vi "test Process Records.vi"(8 "error in":errorcluster, 11 "TestCase in":refnum<class "Engine.lvclass">) -> (0 "error out":errorcluster, 3 "TestCase out":refnum<class "Engine.lvclass">)   [LabVIEW 2023, in "Engine.lvclass"]
uses:
  Engine.lvclass
  Engine.lvclass/Engine.ctl
  <vilib>/addons/_JKI Toolkits/VI Tester/TestCase.llb/TestCase.lvclass
  <instrlib>/BTICardLib/Public/Controls/429 Record.ctl
  <instrlib>/BTICardLib/BTICardLV.lvlib
  <vilib>/NI VeriStand/Custom Device API/Data Reference.ctl
  <vilib>/NI VeriStand/Custom Device API/Custom Device API.lvlib
  <vilib>/NI VeriStand/Custom Device API/Custom Device Item Ref.ctl
  Shared/Transfer Type.ctl
  <vilib>/NI/NI VeriStand Encoding and Decoding/Encoding.ctl
  <vilib>/NI/NI VeriStand Encoding and Decoding/Encoding and Decoding.lvlib
  Shared/Parameter Definition.ctl
  Shared/RT Parameters.ctl
  Shared/Label.ctl
  Shared/RT Label Settings.ctl
  Shared/RT Hardware Channel Settings.ctl
  Shared/Map of Identifiers to Indexes.ctl
  Engine/Custom Device/Custom Device.lvlib
  C:/Program Files/National Instruments/LabVIEW 2023/vi.lib/addons/_JKI Toolkits/VI Tester/TestCase.llb/TestCase.lvclass
  C:/dev/niveristand-ballard-arinc429-custom-device/Source/Custom Device Support/Tests/Unit/Execution/Engine/Engine.lvclass
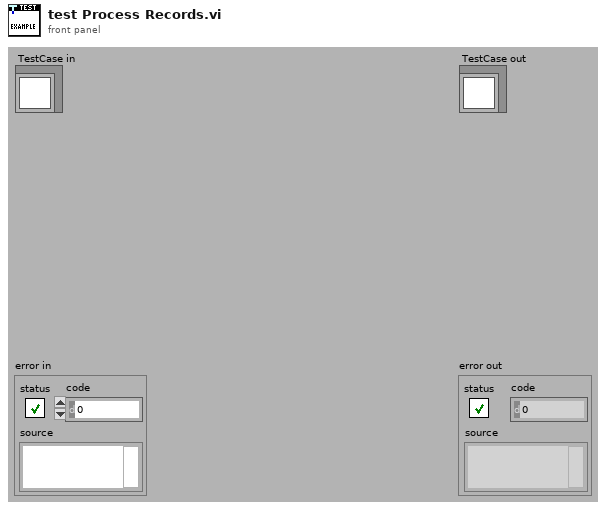
[diagram p1: front panel]
types:
  T1 = typedef "Map of Identifiers to Indexes.ctl" = map{u32, cluster{"channel index":i32, "label index":i32, "start index":i32, "parameters":i32, "timestamp index":i32}}
  T2 = typedef "BTICardLV.lvlib/429 Record.ctl" = cluster{"type":u16, "count":u16, "timestamp":u32, "msgact":u16, "decgap":u16, "data":u32, "timestamph":u32}
  T3 = typedef "RT Hardware Channel Settings.ctl" = cluster{"channel #":u16, "channel handle":u64, "labels settings for RT":T4[]}
  T4 = typedef "RT Label Settings.ctl" = cluster{"Name":string, "xmlName":string, "label":T5, "transfer period":u32, "SDI_Enabled":bool, "SDI":u8, "parameter driver data":T6, "transfer type":T10, "has timestamp?":bool, "Label Disable/Trigger Channel Reference":T9, "Message Handle":u64, "Initialized?":bool, "Word Initial Raw Value":u32, "Label Timestamp Channel Data Reference":T11, "disabled":bool}
  T5 = typedef "Label.ctl" = u8
  T6 = typedef "RT Parameters.ctl" = cluster{"parameter definitions":T7[], "Tx parameter refs":T9[]}
  T7 = typedef "Parameter Definition.ctl" = cluster{"start index":i32, "size":i32, "encoding":T8, "signed":bool, "scale multiplier":dbl, "scale offset":dbl}
  T8 = typedef "Encoding and Decoding.lvlib/Encoding.ctl" = enum16{"BNR", "BCD", "Discrete"}
  T9 = typedef "Custom Device API.lvlib/Custom Device Item Ref.ctl" = u64
  T10 = typedef "Transfer Type.ctl" = enum16{"Scheduled", "Acyclic", "Block", "Strobe"}
  T11 = typedef "Custom Device API.lvlib/Data Reference.ctl" = i32
  T12 = cluster{"message info":u32, "data word":u32, "timestamp":dbl}
  T13 = cluster{"channel index":i32, "label index":i32, "start index":i32, "parameters":i32, "timestamp index":i32}[]
  T14 = cluster{"message info":u32, "data word":u32, "timestamp":dbl}[]
  T15 = cluster{"hardware channel":u8, "label":u8, "SDI":u8}
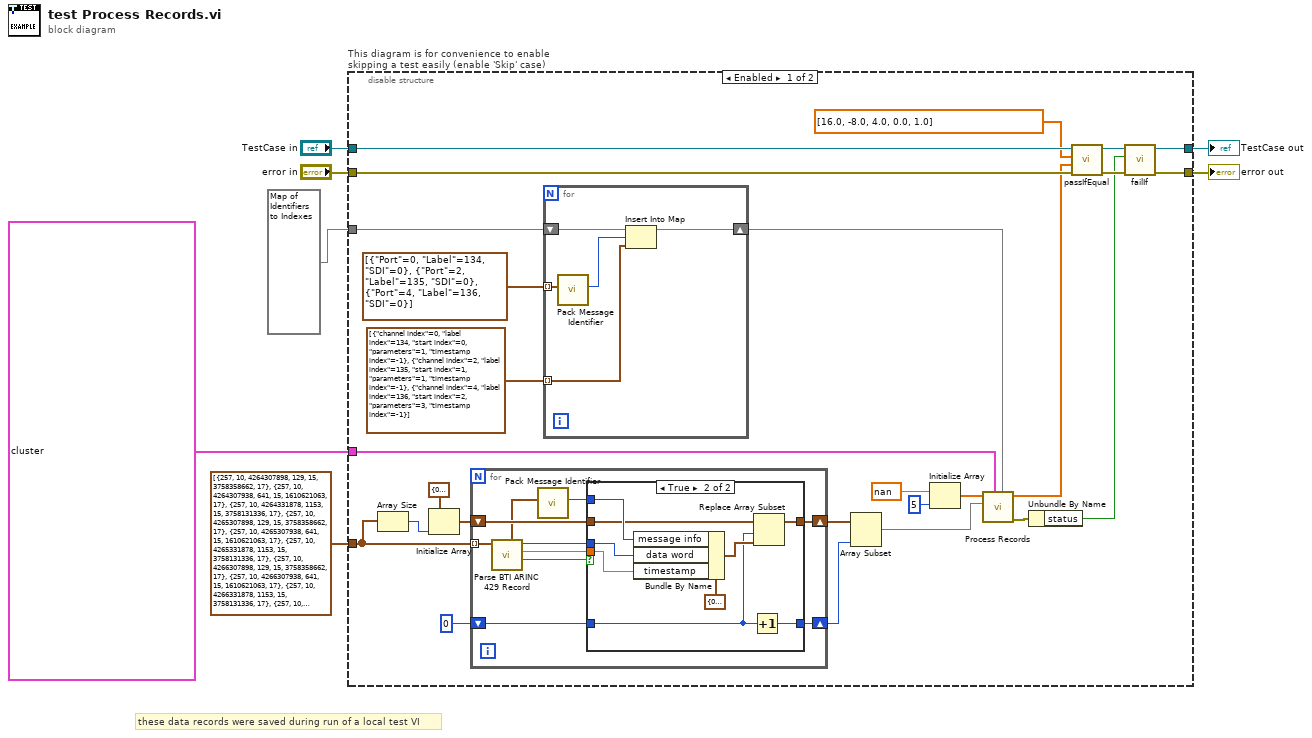
[diagram p0: block diagram]
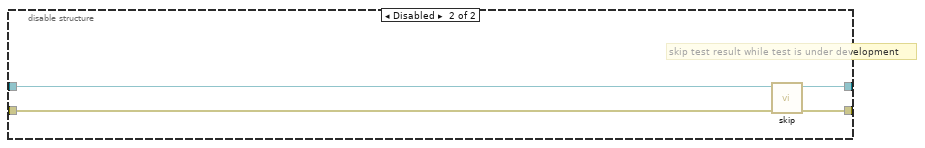
[diagram p3: hidden frame]
diagram:
  # "these data records were saved during run of a local test VI"
  n1 = disable-structure "This diagram is for convenience to enable skipping a test easily (enable 'Skip' case)" shown="Enabled" {
    disable-tunnel: "TestCase in" -> [w29 w63]
    disable-tunnel: [w33 w61] -> w4
    disable-tunnel: [w32 w62] -> w6
    disable-tunnel: "error in" -> [w28 w60]
    disable-tunnel: T3[] data[160728B] ("RT hardware channel data") -> [w20 _]
    disable-tunnel: T2[] [{"type"=257, "count"=10, "timestamp"=4264307898, "msgact"=129, "decgap"=15, "data"=3758358662, "timestamph"=17}, {"type"=257, "count"=10, "timestamp"=4264307938, "msgact"=641, "decgap"=15, "data"=1610621063, "timestamph"=17}, {"type"=257, "count"=10, "timestamp"=4264331878, "msgact"=1153, "decgap"=15, "data"=3758131336, "timestamph"=17}, {"type"=257, "count"=10, "timestamp"=4265307898, "msgact"=129, "decgap"=15, "data"=3758358662, "timestamph"=17}, {"type"=257, "count"=10, "timestamp"=4265307938, "msgact"=641, "decgap"=15, "data"=1610621063, "timestamph"=17}, {"type"=257, "count"=10, "timestamp"=4265331878, "msgact"=1153, "decgap"=15, "data"=3758131336, "timestamph"=17}, {"type"=257, "count"=10, "timestamp"=4266307898, "msgact"=129, "decgap"=15, "data"=3758358662, "timestamph"=17}, {"type"=257, "count"=10, "timestamp"=4266307938, "msgact"=641, "decgap"=15, "data"=1610621063, "timestamph"=17}, {"type"=257, "count"=10, "timestamp"=4266331878, "msgact"=1153, "decgap"=15, "data"=3758131336, "timestamph"=17}, {"type"=257, "count"=10, "timestamp"=4267307898, "msgact"=129, "decgap"=15, "data"=3758358662, "timestamph"=17}, {"type"=257, "count"=10, "timestamp"=4267307938, "msgact"=641, "decgap"=15, "data"=1610621063, "timestamph"=17}, {"type"=257, "count"=10, "timestamp"=4267331858, "msgact"=1153, "decgap"=15, "data"=3758131336, "timestamph"=17}, {"type"=257, "count"=10, "timestamp"=4268307898, "msgact"=129, "decgap"=15, "data"=3758358662, "timestamph"=17}, {"type"=257, "count"=10, "timestamp"=4268307938, "msgact"=641, "decgap"=15, "data"=1610621063, "timestamph"=17}, {"type"=257, "count"=10, "timestamp"=4268331858, "msgact"=1153, "decgap"=15, "data"=3758131336, "timestamph"=17}, {"type"=257, "count"=10, "timestamp"=4269307898, "msgact"=129, "decgap"=15, "data"=3758358662, "timestamph"=17}, {"type"=257, "count"=10, "timestamp"=4269307938, "msgact"=641, "decgap"=15, "data"=1610621063, "timestamph"=17}, {"type"=257, "count"=10, "timestamp"=4269331858, "msgact"=1153, "decgap"=15, "data"=3758131336, "timestamph"=17}, {"type"=257, "count"=10, "timestamp"=4270307898, "msgact"=129, "decgap"=15, "data"=3758358662, "timestamph"=17}, {"type"=257, "count"=10, "timestamp"=4270307938, "msgact"=641, "decgap"=15, "data"=1610621063, "timestamph"=17}, {"type"=257, "count"=10, "timestamp"=4270331878, "msgact"=1153, "decgap"=15, "data"=3758131336, "timestamph"=17}, {"type"=257, "count"=10, "timestamp"=4271307898, "msgact"=129, "decgap"=15, "data"=3758358662, "timestamph"=17}, {"type"=257, "count"=10, "timestamp"=4271307938, "msgact"=641, "decgap"=15, "data"=1610621063, "timestamph"=17}, {"type"=257, "count"=10, "timestamp"=4271331858, "msgact"=1153, "decgap"=15, "data"=3758131336, "timestamph"=17}, {"type"=257, "count"=10, "timestamp"=4272307898, "msgact"=129, "decgap"=15, "data"=3758358662, "timestamph"=17}, {"type"=257, "count"=10, "timestamp"=4272307938, "msgact"=641, "decgap"=15, "data"=1610621063, "timestamph"=17}, {"type"=257, "count"=10, "timestamp"=4272331858, "msgact"=1153, "decgap"=15, "data"=3758131336, "timestamph"=17}, {"type"=257, "count"=10, "timestamp"=4273307898, "msgact"=129, "decgap"=15, "data"=3758358662, "timestamph"=17}, {"type"=257, "count"=10, "timestamp"=4273307938, "msgact"=641, "decgap"=15, "data"=1610621063, "timestamph"=17}, {"type"=257, "count"=10, "timestamp"=4273331878, "msgact"=1153, "decgap"=15, "data"=3758131336, "timestamph"=17}, {"type"=257, "count"=10, "timestamp"=4274307898, "msgact"=129, "decgap"=15, "data"=3758358662, "timestamph"=17}, {"type"=257, "count"=10, "timestamp"=4274307938, "msgact"=641, "decgap"=15, "data"=1610621063, "timestamph"=17}, {"type"=257, "count"=10, "timestamp"=4274331858, "msgact"=1153, "decgap"=15, "data"=3758131336, "timestamph"=17}, {"type"=257, "count"=10, "timestamp"=4275307898, "msgact"=129, "decgap"=15, "data"=3758358662, "timestamph"=17}, {"type"=257, "count"=10, "timestamp"=4275307938, "msgact"=641, "decgap"=15, "data"=1610621063, "timestamph"=17}, {"type"=257, "count"=10, "timestamp"=4275331858, "msgact"=1153, "decgap"=15, "data"=3758131336, "timestamph"=17}, {"type"=257, "count"=10, "timestamp"=4276307898, "msgact"=129, "decgap"=15, "data"=3758358662, "timestamph"=17}, {"type"=257, "count"=10, "timestamp"=4276307938, "msgact"=641, "decgap"=15, "data"=1610621063, "timestamph"=17}, {"type"=257, "count"=10, "timestamp"=4276331858, "msgact"=1153, "decgap"=15, "data"=3758131336, "timestamph"=17}, {"type"=257, "count"=10, "timestamp"=4277307898, "msgact"=129, "decgap"=15, "data"=3758358662, "timestamph"=17}, {"type"=257, "count"=10, "timestamp"=4277307938, "msgact"=641, "decgap"=15, "data"=1610621063, "timestamph"=17}, {"type"=257, "count"=10, "timestamp"=4277331858, "msgact"=1153, "decgap"=15, "data"=3758131336, "timestamph"=17}] ("records") -> [w14 _]
    disable-tunnel: T1 {} ("map from message info to indexes") -> [w19 _]
    frame Enabled {
      n2 = Array Size(array=w14) -> (size(s)=w12:i32)
      n3 = Initialize Array(T12 {"message info"=0, "data word"=0, "timestamp"=0.0}, w12) -> (w13:T14)
      n4 = for {
        tunnel: w14 -> [w43] mode=indexing
        shift-right: [w40] -> w10
        shift-left: w13 -> [w41]
        shift-right: [w34] -> w9
        shift-left: 0 -> [w35]
        n5 = call "Parse BTI ARINC 429 Record.vi"("record"=w43) -> ("hit"=w38:bool, "time stamp"=w42:dbl, "data word"=w39:u32, "message info"=w37:T15)  [unwired: 5 in, 2 out]
        n6 = call "Pack Message Identifier.vi"("message identifiers"=w37) -> ("packed message identifier"=w36:u32)  [unwired: 10 in]
        n7 = case shown="True" w38 {
          tunnel: w41 -> [w45 w47]
          tunnel: [w45 w46] -> w40
          tunnel: w36 -> [_ w52]
          tunnel: w39 -> [_ w51]
          tunnel: w42 -> [_ w50]
          tunnel: w35 -> [w44 w48]
          tunnel: [w44 w49] -> w34
          frame False {
          }
          frame True {
            n8 = Bundle By Name(cluster=T12 {"message info"=0, "data word"=0, "timestamp"=0.0}, "message info"=w52, "data word"=w51, "timestamp"=w50) -> (w53:T12)
            n9 = Increment(x=w48) -> (x+1=w49:i32)
            n10 = Replace Array Subset(array=w47, new element=w53, index=w48) -> (w46:T14)
          }
        }
      }
      n11 = for {
        shift-right: [w55] -> w16
        shift-left: w19 -> [w59]
        tunnel: cluster{"Port":u8, "Label":u8, "SDI":u8}[] [{"Port"=0, "Label"=134, "SDI"=0}, {"Port"=2, "Label"=135, "SDI"=0}, {"Port"=4, "Label"=136, "SDI"=0}] -> [w58] mode=indexing
        tunnel: T13 [{"channel index"=0, "label index"=134, "start index"=0, "parameters"=1, "timestamp index"=-1}, {"channel index"=2, "label index"=135, "start index"=1, "parameters"=1, "timestamp index"=-1}, {"channel index"=4, "label index"=136, "start index"=2, "parameters"=3, "timestamp index"=-1}] -> [w56] mode=indexing
        n12 = call "Pack Message Identifier.vi"("message identifiers"=w58) -> ("packed message identifier"=w57:u32)  [unwired: 10 in]
        n13 = Insert Into Map(map in=w59, key=w57, value=w56) -> (map out=w55:T1)  [unwired: 2 out]
      }
      n14 = Array Subset(array=w10, length=w9) -> (w8:T14)  [unwired: 1 in]
      n15 = Initialize Array(nan ("element"), 5 ("dimension size")) -> (w23:dbl[])
      n16 = call "Process Records.vi"("map from message info to indexes"=w16, "RT hardware channel data"=w20, "map of message info to data word"=w8, "parameter values in"=w23) -> ("error out"=w27:errorcluster, "parameter values out"=w22:dbl[])  [unwired: 4 in]
      n17 = Unbundle By Name(w27) -> ("status"=w26:bool)
      n18 = call-dynamic "passIfEqual.vi"("error in (no error)"=w28, "y"=w22, "x"=dbl[] [16.0, -8.0, 4.0, 0.0, 1.0] ("parameter values out"), "TestCase in"=w29) -> ("error out"=w30:errorcluster, "TestCase out"=w31:refnum<class "Engine.lvclass">)  [unwired: 6 in]
      n19 = call-dynamic "failIf.vi"("error in (no error)"=w30, "fail"=w26, "TestCase in"=w31) -> ("error out"=w32:errorcluster, "TestCase out"=w33:refnum<class "Engine.lvclass">)  [unwired: 7 in]
    }
    frame Disabled {
      # "skip test result while test is under development"
      n20 = call <vilib>:"skip.vi"("error in (no error)"=w60, "TestCase in"=w63) -> ("error out"=w62:errorcluster, "TestCase out"=w61:refnum<class "Engine.lvclass">)  [unwired: 8 in]
    }
  }
  "error out" <- w6
  "TestCase out" <- w4
